vi "MGI Bezier Build Initial Simplex.vi"(0 "Start[]":dbl[](array[numeric]) format="%.2f") -> (1 "Minimum before[][]":dbl[][](array[numeric]) format="%.2f", 2 "f(Minimum) before[]":dbl[](array[numeric]) format="%.2f")   [LabVIEW 2016]
doc: "Part of LabVIEW code that defines the initial simplex. Spacing is 10% in each dimension, or +1 if the value is zero. That's different than the normal LabVIEW technique.\n\nAuthored by David A. Moore\nsupport@mooregoodideas.com\nwww.mooregoodideas.com\n\nCopyright (c) 2010, Moore Good Ideas, Inc.\n\nAll rights reserved.\n\nRedistribution and use in source and binary forms, with or without modification, are permitted provided that the following conditions are met:\n\n * Redistributions of source code must retain the above copyright notice, this list of conditions and the following disclaimer.\n * Redistributions in binary form must reproduce the above copyright notice, this list of conditions and the following disclaimer in the documentation and/or other materials provided with the distribution.\n * Neither the name of Moore Good Ideas, Inc. nor the names of its contributors may be used to endorse or promote products derived from this software without specific prior written permission.\n\nTHIS SOFTWARE IS PROVIDED BY THE COPYRIGHT HOLDERS AND CONTRIBUTORS \"AS IS\" AND ANY EXPRESS OR IMPLIED WARRANTIES, INCLUDING, BUT NOT LIMITED TO, THE IMPLIED WARRANTIES OF MERCHANTABILITY AND FITNESS FOR A PARTICULAR PURPOSE ARE DISCLAIMED. IN NO EVENT SHALL THE COPYRIGHT OWNER OR CONTRIBUTORS BE LIABLE FOR ANY DIRECT, INDIRECT, INCIDENTAL, SPECIAL, EXEMPLARY, OR CONSEQUENTIAL DAMAGES (INCLUDING, BUT NOT LIMITED TO, PROCUREMENT OF SUBSTITUTE GOODS OR SERVICES; LOSS OF USE, DATA, OR PROFITS; OR BUSINESS INTERRUPTION) HOWEVER CAUSED AND ON ANY THEORY OF LIABILITY, WHETHER IN CONTRACT, STRICT LIABILITY, OR TORT (INCLUDING NEGLIGENCE OR OTHERWISE) ARISING IN ANY WAY OUT OF THE USE OF THIS SOFTWARE, EVEN IF ADVISED OF THE POSSIBILITY OF SUCH DAMAGE."
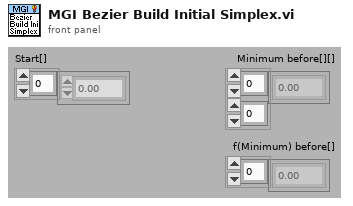
[diagram p1: front panel]
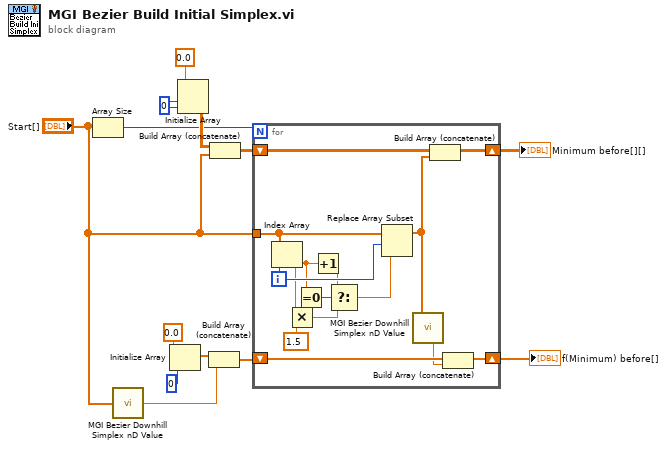
[diagram p0: block diagram]
diagram:
  w7 = 0
  n1 = Array Size(array="Start[]") -> (size(s)=w8:i32)
  n2 = call <userlib>:"MGI Bezier Downhill Simplex nD Value.vi"("x[]"="Start[]") -> ("f(x)"=w3:dbl)
  n3 = Initialize Array(0.0, 0) -> (w4:dbl[])
  n4 = Initialize Array(0.0, w7, w7) -> (w10:dbl[][])
  n5 = Build Array (concatenate)(w4, w3) -> (w2:dbl[])
  n6 = Build Array (concatenate)(w10, "Start[]") -> (w9:dbl[][])
  n7 = for {
    N: w8 -> [_]
    shift-right: [w26] -> w13
    shift-left: w9 -> [w27]
    shift-right: [w24] -> w12
    shift-left: w2 -> [w25]
    tunnel: "Start[]" -> [w21]
    i -> [w22]
    n8 = Index Array(array=w21, index=w22) -> (element=w16:dbl)
    n9 = Multiply(x=w16, y=1.5) -> (x*y=w15:dbl)
    n10 = Equal To 0?(x=w16) -> (x = 0?=w19:bool)
    n11 = Increment(x=w16) -> (x+1=w18:dbl)
    n12 = Select(t=w18, s=w19, f=w15) -> (s? t:f=w17:dbl)
    n13 = Replace Array Subset(array=w21, new element=w17, index=w22) -> (w20:dbl[])
    n14 = call <userlib>:"MGI Bezier Downhill Simplex nD Value.vi"("x[]"=w20) -> ("f(x)"=w23:dbl)
    n15 = Build Array (concatenate)(w27, w20) -> (w26:dbl[][])
    n16 = Build Array (concatenate)(w25, w23) -> (w24:dbl[])
  }
  "Minimum before[][]" <- w13
  "f(Minimum) before[]" <- w12
